vi "determine necessary types and order.vi"(10 "supported types":T1[](array[typedef]), 11 "dictionary":T2) -> (3 "output type order":T1[](array[typedef]))   [LabVIEW 2013, in "TDMS datalogger runtime.lvclass"]
uses:
  TDMS datalogger runtime.lvclass
  <vilib>/NI/Tag Bus/tag/Data Type.ctl
  <vilib>/NI/Tag Bus/dictionary/full data dictionary.ctl
  <vilib>/NI/Tag Bus/tag/tag descriptor.lvclass
  <vilib>/NI/Tag Bus/dictionary/data dictionary.lvclass
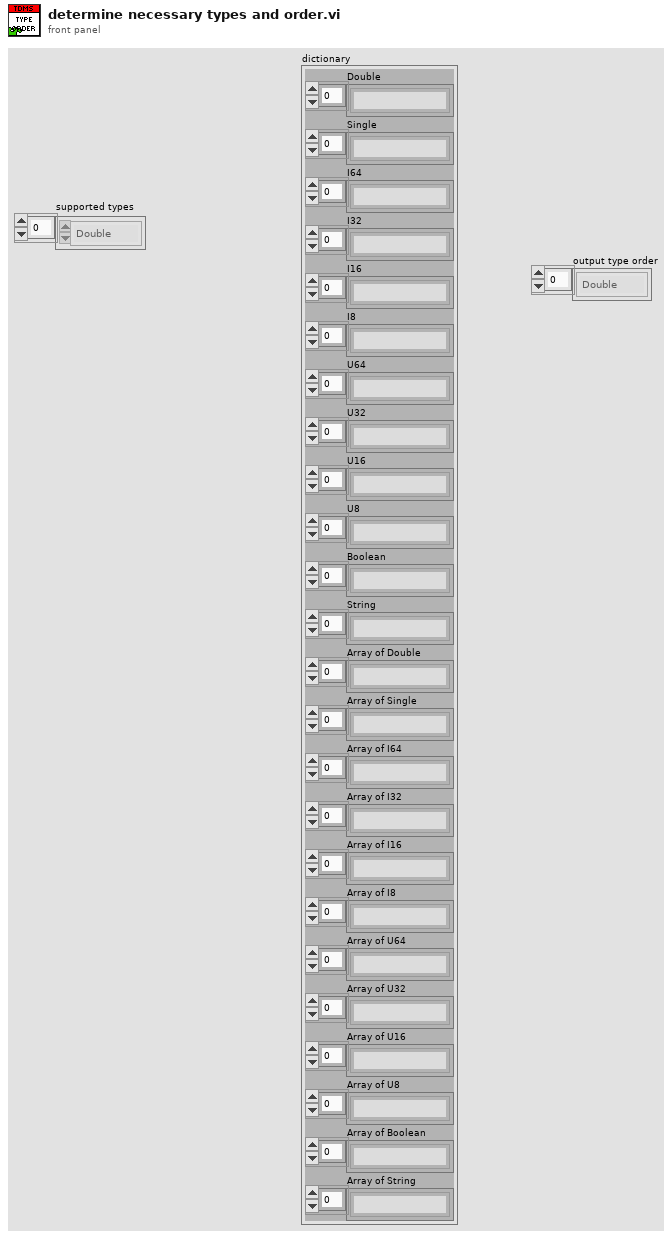
[diagram p1: front panel]
types:
  T1 = typedef "tag bus.lvlib/tag descriptor.lvclass/Data Type.ctl" = enum16{"Double", "Single", "I64", "I32", "I16", "I8", "U64", "U32", "U16", "U8", "Boolean", "String", "Array of Double", "Array of Single", "Array of I64", "Array of I32", "Array of I16", "Array of I8", "Array of U64", "Array of U32", "Array of U16", "Array of U8", "Array of Boolean", "Array of String"}
  T2 = typedef "tag bus.lvlib/data dictionary.lvclass/full data dictionary.ctl" = cluster{"Double":string[], "Single":string[], "I64":string[], "I32":string[], "I16":string[], "I8":string[], "U64":string[], "U32":string[], "U16":string[], "U8":string[], "Boolean":string[], "String":string[], "Array of Double":string[], "Array of Single":string[], "Array of I64":string[], "Array of I32":string[], "Array of I16":string[], "Array of I8":string[], "Array of U64":string[], "Array of U32":string[], "Array of U16":string[], "Array of U8":string[], "Array of Boolean":string[], "Array of String":string[]}
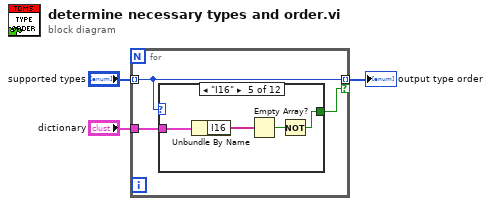
[diagram p0: block diagram]
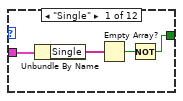
[diagram p2: hidden frame]
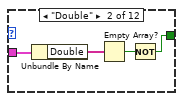
[diagram p3: hidden frame]
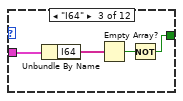
[diagram p4: hidden frame]
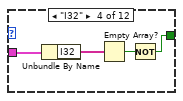
[diagram p5: hidden frame]
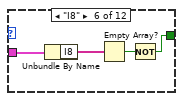
[diagram p6: hidden frame]
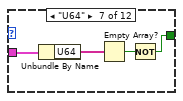
[diagram p7: hidden frame]
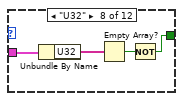
[diagram p8: hidden frame]
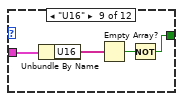
[diagram p9: hidden frame]
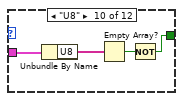
[diagram p10: hidden frame]
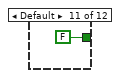
[diagram p11: hidden frame]
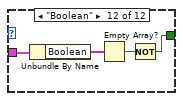
[diagram p12: hidden frame]
diagram:
  n1 = for {
    tunnel: "dictionary" -> [w5]
    tunnel: "supported types" -> [w6] mode=indexing
    tunnel: [w6] -> w1 mode=indexing if=w4
    n2 = case shown="\"I16\"" w6 {
      tunnel: w5 -> [w9 w13 w17 w21 w25 w29 w34 w37 w41 w45 _ w50]
      tunnel: [w7 w12 w16 w20 w24 w28 w31 w36 w39 w44 FALSE w49] -> w4
      frame "Single" {
        n3 = Unbundle By Name(w9) -> ("Single"=w8:string[])
        n4 = Empty Array?(array=w8) -> (empty?=w10:bool)
        n5 = Not(x=w10) -> (.not. x?=w7:bool)
      }
      frame "Double" {
        n6 = Unbundle By Name(w13) -> ("Double"=w11:string[])
        n7 = Empty Array?(array=w11) -> (empty?=w14:bool)
        n8 = Not(x=w14) -> (.not. x?=w12:bool)
      }
      frame "I64" {
        n9 = Unbundle By Name(w17) -> ("I64"=w15:string[])
        n10 = Empty Array?(array=w15) -> (empty?=w18:bool)
        n11 = Not(x=w18) -> (.not. x?=w16:bool)
      }
      frame "I32" {
        n12 = Unbundle By Name(w21) -> ("I32"=w19:string[])
        n13 = Empty Array?(array=w19) -> (empty?=w22:bool)
        n14 = Not(x=w22) -> (.not. x?=w20:bool)
      }
      frame "I16" {
        n15 = Unbundle By Name(w25) -> ("I16"=w23:string[])
        n16 = Empty Array?(array=w23) -> (empty?=w26:bool)
        n17 = Not(x=w26) -> (.not. x?=w24:bool)
      }
      frame "I8" {
        n18 = Unbundle By Name(w29) -> ("I8"=w27:string[])
        n19 = Empty Array?(array=w27) -> (empty?=w30:bool)
        n20 = Not(x=w30) -> (.not. x?=w28:bool)
      }
      frame "U64" {
        n21 = Unbundle By Name(w34) -> ("U64"=w33:string[])
        n22 = Empty Array?(array=w33) -> (empty?=w32:bool)
        n23 = Not(x=w32) -> (.not. x?=w31:bool)
      }
      frame "U32" {
        n24 = Unbundle By Name(w37) -> ("U32"=w35:string[])
        n25 = Empty Array?(array=w35) -> (empty?=w38:bool)
        n26 = Not(x=w38) -> (.not. x?=w36:bool)
      }
      frame "U16" {
        n27 = Unbundle By Name(w41) -> ("U16"=w40:string[])
        n28 = Empty Array?(array=w40) -> (empty?=w42:bool)
        n29 = Not(x=w42) -> (.not. x?=w39:bool)
      }
      frame "U8" {
        n30 = Unbundle By Name(w45) -> ("U8"=w43:string[])
        n31 = Empty Array?(array=w43) -> (empty?=w46:bool)
        n32 = Not(x=w46) -> (.not. x?=w44:bool)
      }
      frame Default {
      }
      frame "Boolean" {
        n33 = Unbundle By Name(w50) -> ("Boolean"=w48:string[])
        n34 = Empty Array?(array=w48) -> (empty?=w51:bool)
        n35 = Not(x=w51) -> (.not. x?=w49:bool)
      }
    }
  }
  "output type order" <- w1
